vi "AcuurDataOut.vi"(8 "error in (no error)":errorcluster, 10 "通道":u16(ring) items=["直流CH1", "直流CH2", "直流CH3", "直流CH4", "直流CH5", "直流CH6", "直流CH7", "直流CH8", "直流CH9", "直流CH10"], 11 "测试类型":string) -> (0 "error out 2":errorcluster, 3 "表格控件 2":string[][](table))   [LabVIEW 2014]
uses:
  <vilib>/addons/database/Connection.llb/DB Tools Open Connec (String).vi
  <vilib>/addons/database/Connection.llb/Conn Execute.vi
  <vilib>/addons/database/Recordset.llb/Rec Fetch Recordset Data (R).vi
  <vilib>/addons/database/Recordset.llb/Rec Destroy - Connection.vi
  <vilib>/addons/database/_DB Variant To Data/Database Variant To Data.xnode
  <vilib>/addons/database/NI_Database_API.lvlib
panel:
  in  "测试类型":u16(ring) items=["温循", "高温老练", "常温拷机", "自定义测试", "单次测试", "自动测试"]
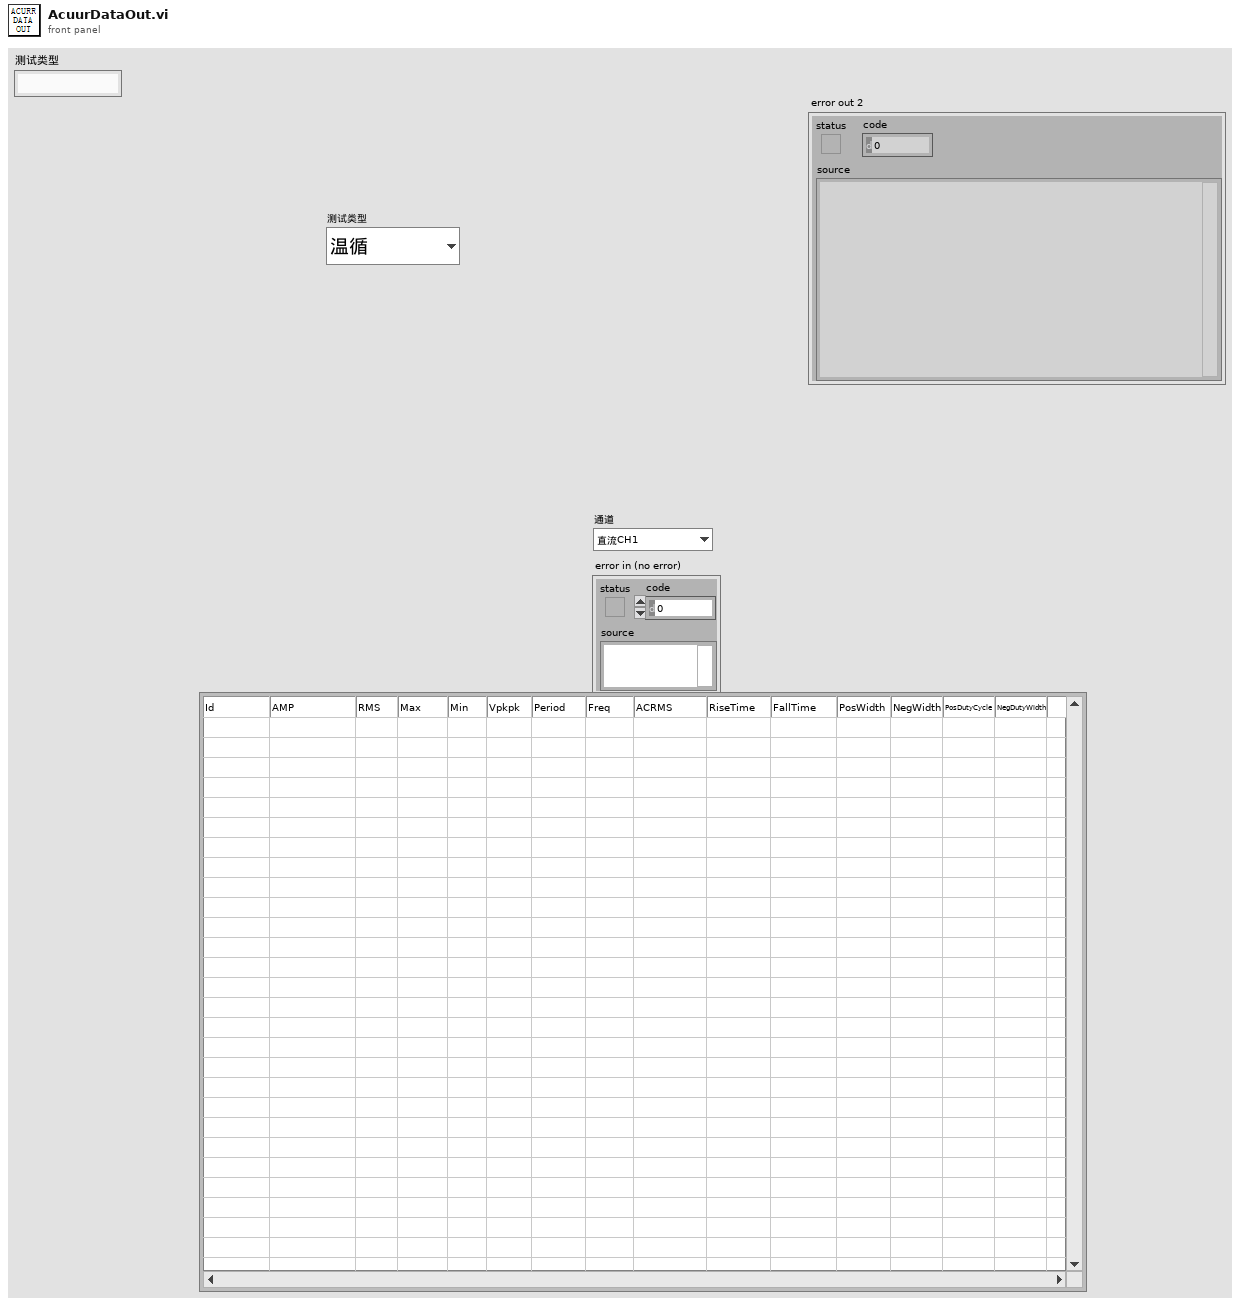
[diagram p1: front panel]
types:
  T1 = typedef "NI_Database_API.lvlib/Conn ObjectReference.ctl" = refnum<k1>
  T2 = typedef "NI_Database_API.lvlib/Rec ObjectReference.ctl" = refnum<k1>
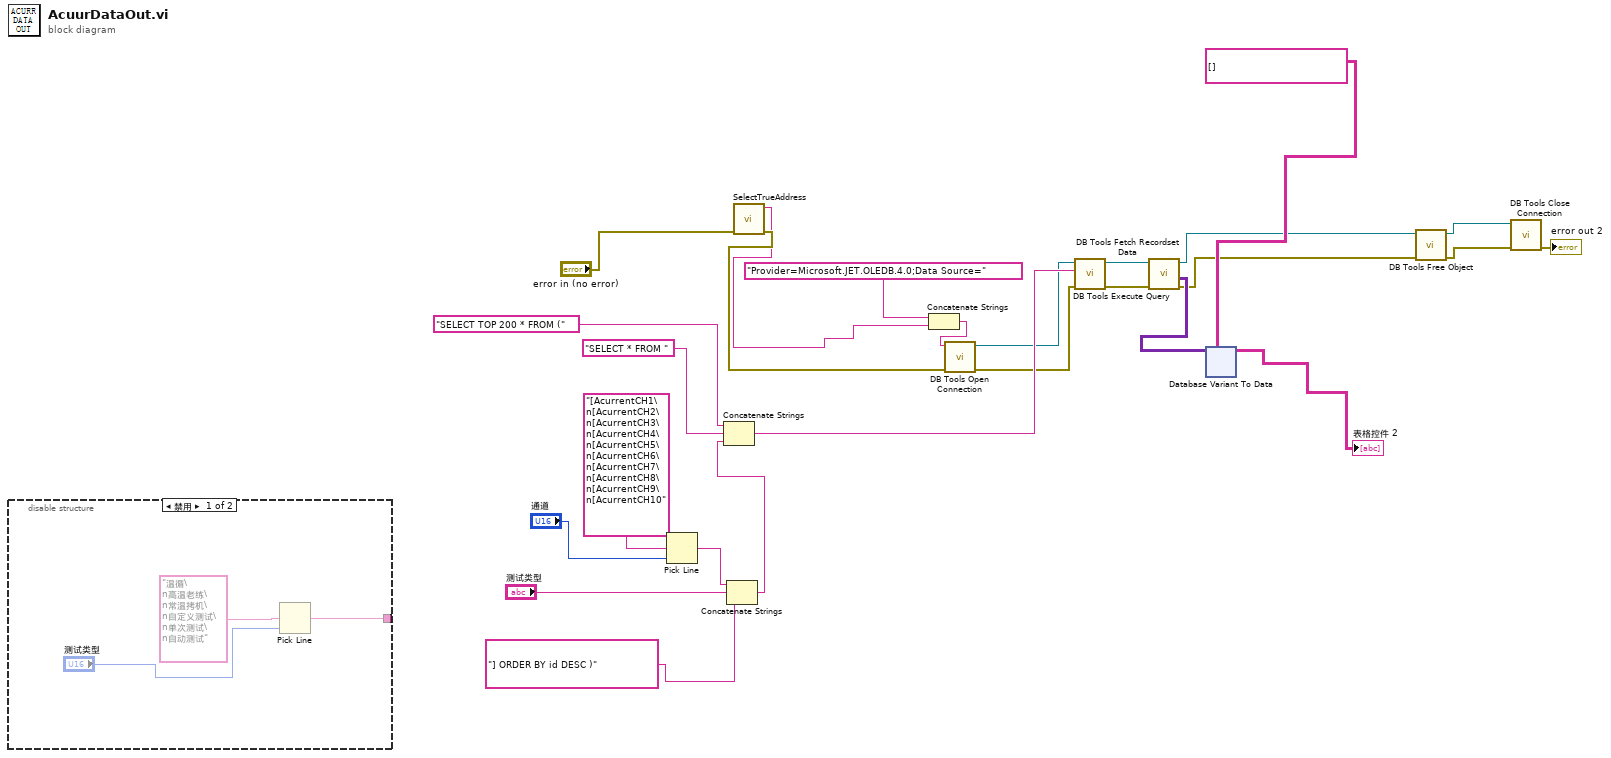
[diagram p0: block diagram]
diagram:
  n1 = disable-structure shown="禁用" {
    disable-tunnel: [w29 _] -> _
    frame Disabled {
      n2 = Pick Line(multi-line string="温循\n高温老练\n常温拷机\n自定义测试\n单次测试\n自动测试" ("多行字符串"), line index="测试类型") -> (output string=w29:string)  [unwired: 1 in]
    }
    frame Enabled {
    }
  }
  n3 = Pick Line(multi-line string="[AcurrentCH1\n[AcurrentCH2\n[AcurrentCH3\n[AcurrentCH4\n[AcurrentCH5\n[AcurrentCH6\n[AcurrentCH7\n[AcurrentCH8\n[AcurrentCH9\n[AcurrentCH10" ("多行字符串"), line index="通道") -> (output string=w9:string)  [unwired: 1 in]
  n4 = Concatenate Strings(w9, "测试类型", "] ORDER BY id DESC )") -> (w10:string)
  n5 = Concatenate Strings("SELECT TOP 200 * FROM (" ("字符串"), "SELECT * FROM ", w10) -> (w25:string)
  n6 = call "SelectTrueAddress.vi"("error in (no error)"="error in (no error)") -> ("error out"=w22:errorcluster, "元素"=w20:string)  [unwired: 9 in]
  n7 = Concatenate Strings("Provider=Microsoft.JET.OLEDB.4.0;Data Source=", w20) -> (w21:string)
  n8 = call-poly <vilib>:"DB Tools Open Connection.vi"("error in (no error)"=w22, "connection information"=w21) -> ("error out"=w24:errorcluster, "connection reference"=w23:T1)  [unwired: 6 in]
  n9 = call-poly <vilib>:"DB Tools Execute Query.vi"("error in (no error)"=w24, "SQL query"=w25, "connection reference"=w23) -> ("error out"=w15:errorcluster, "recordset reference"=w14:T2)  [unwired: 5 in]
  n10 = call-poly <vilib>:"DB Tools Fetch Recordset Data.vi"("error in (no error)"=w15, "recordset reference"=w14) -> ("error out"=w17:errorcluster, "recordset data"=w26:variant[][], "recordset reference out"=w16:T2)  [unwired: 3 in]
  n11 = xnode "Database Variant To Data"("database variant"=w26, "type"=string[][] []) -> ("data"=→"表格控件 2":string[][])  [unwired: 1 in, 1 out]
  n12 = call-poly <vilib>:"DB Tools Free Object.vi"("error in (no error)"=w17, "recordset reference"=w16) -> ("error out"=w12:errorcluster, "connection reference"=w13:T1)  [unwired: 8 in]
  n13 = call <vilib>:"DB Tools Close Connection.vi"("error in (no error)"=w12, "connection reference"=w13) -> ("error out"=→"error out 2":errorcluster)  [unwired: 5 in]
